vi "Value Multiple Boolean Controls.vi"(8 "error in":errorcluster, 10 "Value":bool, 11 "References":refnum<vi>[](array[refnum])) -> (0 "error out":errorcluster)   [LabVIEW 2015]
doc: "Sets TRUE or FALSE value for a group of Boolean controls"
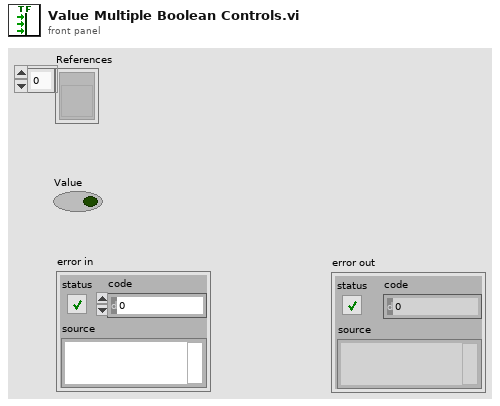
[diagram p1: front panel]
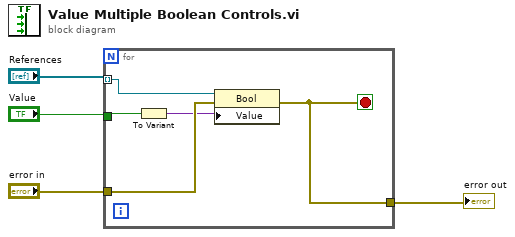
[diagram p0: block diagram]
diagram:
  n1 = for {
    tunnel: "References" -> [w9] mode=indexing
    tunnel: "Value" -> [w6]
    tunnel: "error in" -> [w8]
    tunnel: [w7] -> w1
    stop <- w7 stop-if-true
    n2 = To Variant(anything=w6) -> (Variant=w5:variant)
    n3 = property class="Bool"(reference=w9, error in=w8, "Value"=w5) -> (error out=w7:errorcluster)  [unwired: 1 out]
  }
  "error out" <- w1
